vi "Set units.vi"(7 "[x]":T1, 8 "error in (no error)":errorcluster, 10 "Units":T2, 11 "Serial Port in":refnum<visa-resource-name>) -> (0 "error out":errorcluster, 3 "Serial Port out":refnum<visa-resource-name>)   [LabVIEW 2016, in "Chemyx_Syringe_Pump_driver.lvlib"]
doc: "Set the rate and volume units of the pump. \n\nUnits are defined by an enum with the following items:\n0: ml/min\n1: ml/hr\n2: ul/min\n3: ul/hr."
uses:
  Chemyx_Syringe_Pump_driver.lvlib
  controls/unit_enum.ctl
  _private/Control/Control Mode.ctl
panel:
  # "Set the rate and volume units of the pump. \n\nUnits are defined by an enum with the following items:\n0: ml/min\n1: ml/hr\n2: ul/min\n3: ul/hr."
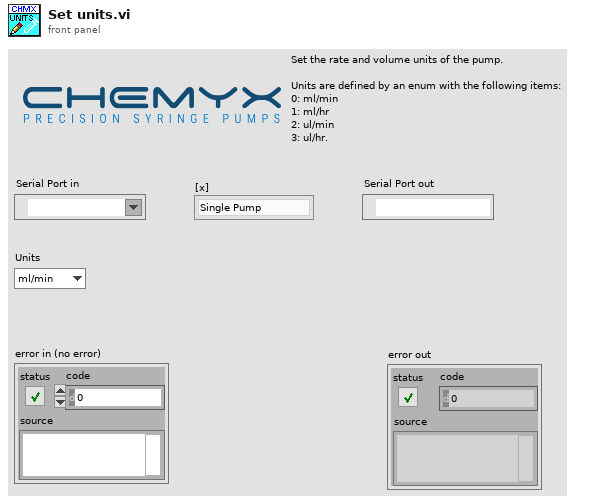
[diagram p1: front panel]
types:
  T1 = typedef "Chemyx_Syringe_Pump_driver.lvlib/Control Mode.ctl" = enum16{"Single Pump", "Pump Chanel 1", "Pump Channel 2", "Cycle Mode"}
  T2 = typedef "Chemyx_Syringe_Pump_driver.lvlib/unit_enum.ctl" = enum16{"ml/min", "ml/hr", "ul/min", "ul/hr"}
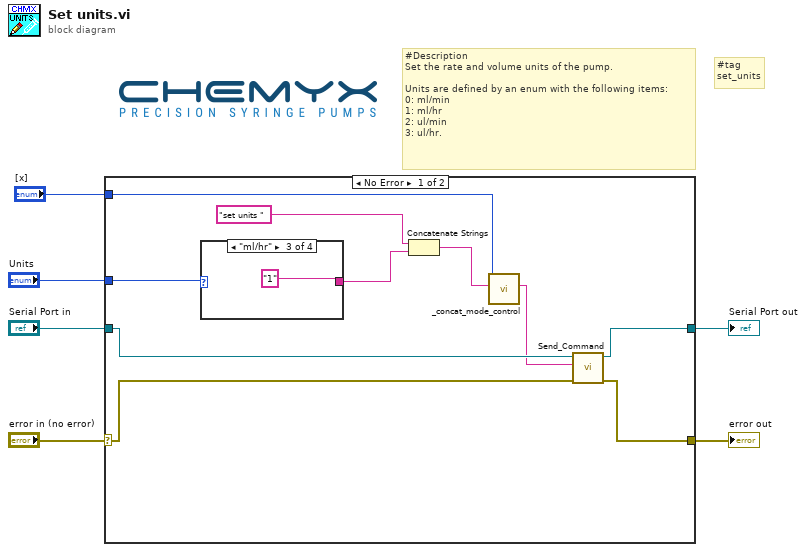
[diagram p0: block diagram]
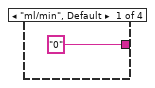
[diagram p2: hidden frame]
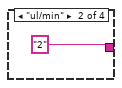
[diagram p3: hidden frame]
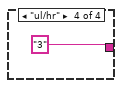
[diagram p4: hidden frame]
diagram:
  # "#tag\nset_units"
  # "#Description\nSet the rate and volume units of the pump. \n\nUnits are defined by an enum with the following items:\n0: ml/min\n1: ml/hr\n2: ul/min\n3: ul/hr."
  n1 = case shown="No Error" "error in (no error)" {
    selector: "error in (no error)" -> [w15 w22]
    tunnel: "Serial Port in" -> [w16 w21]
    tunnel: [w14 w22] -> w4
    tunnel: [w13 w21] -> w3
    tunnel: "Units" -> [w12 _]
    tunnel: "[x]" -> [w7 _]
    frame No Error {
      n2 = case shown="\"ml/hr\"" w12 {
        tunnel: ["0" "2" "1" "3"] -> w10
        frame "ml/min", Default {
        }
        frame "ul/min" {
        }
        frame "ml/hr" {
        }
        frame "ul/hr" {
        }
      }
      n3 = Concatenate Strings("set units ", w10) -> (w9:string)
      n4 = call "_concat_mode_control.vi"("write buffer"=w9, "[x]"=w7) -> ("write buffer out"=w8:string)  [unwired: 9 in]
      n5 = call "Send_Command.vi"("error in (no error)"=w15, "write buffer"=w8, "Serial Port in"=w16) -> ("error out"=w14:errorcluster, "VISA Refnum out"=w13:refnum<visa-resource-name>)  [unwired: 6 in, 1 out]
    }
    frame Error {
    }
  }
  "error out" <- w4
  "Serial Port out" <- w3
